vi "Pendel2.vi"() -> ()   [LabVIEW 2014]
uses:
  Reglertyp.ctl
  <vilib>/Platform/TimedLoop/XDataNode/timing_clust.ctl
  <vilib>/Platform/TimedLoop/XDataNode/nitl_modes.ctl
  <vilib>/Platform/TimedLoop/XDataNode/wakeup.ctl
  <vilib>/Analysis/Matrix/Datatypes/RealMatrix.ctl
  <vilib>/Statechart/Common/IntGuid.ctl
  <vilib>/Statechart/Common/DbgID.ctl
  <vilib>/Analysis/baseanly.llb/Real A x B.vi
  Pendel.lvsc/CompanionDiagram.vi
  Pendel.lvsc/CompanionDiagram.vi/21/SC Main.vi
  Pendel.lvsc/Trigger.ctl
  <vilib>/Statechart/Infrastructure/RTStatechart/RunTime SCN.xnode
  Pendel.lvsc/Inputs.ctl
  Pendel.lvsc/Outputs.ctl
  Pendel.lvsc
  <vilib>/Platform/TimedLoop/XDataNode/XDataNode.xnode
  <vilib>/Platform/TimedLoop/XDataNode/XDNodeRunTimeDep.lvlib
  <vilib>/Analysis/NI_AALBase.lvlib
  <vilib>/Analysis/Matrix/NI_Matrix.lvlib
  <vilib>/ptbypt/NI_PtbyPt.lvlib
  <vilib>/Statechart/Common/NI_SC_LVSCCommonFiles.lvlib
panel:
  out "Kraft berechnet 2":cluster{dbl, dbl, dbl, dbl}(graph)
  out "Winkel 1":dbl
  out "Geschwindigkeit":dbl
  out "Position":dbl
  out "Winkel2":dbl
  out "Winkelgeschwindigkeit2":dbl
  out "Winkelgeschwindigkeit1":dbl
  out "Kraft berechnet":cluster{"Kraft (N)":dbl, dbl}(graph)
  out "Schleifendauer":i64(graph)
  in  "Registerkarte":enum32{"Pendel", "S706", "Wegzähler"}(tab)
  in  "Reglertyp":T1
  in  "Positionieren":bool
  out "Kraft (N)":dbl(graph)
  out "Winkel (Grad)":cluster{"Double":dbl, "Double":dbl}(graph)
  in  "Schließen":bool
  in  "Regler anhalten":bool
  in  "Regler starten":bool
  in  "Ruhelage":bool=TRUE
  in  "Pendelaufbau":T2(ring)
  out "Aktueller Zustand":string
  in  "Referenzieren":bool
  in  "Sollposition (mm)":dbl(slide) scale=-500.0..500.0
  out "Position (mm)":T3(graph)
  out "S706 Status (SDO 6041)":T4
  in  "S706 parametrieren":bool
  out "S706":string
  out "Wegzähler (m)":dbl
  out "Wegzähler (m)":dbl(knob)=6.6072914947233965 scale=5000.0..5000000.0
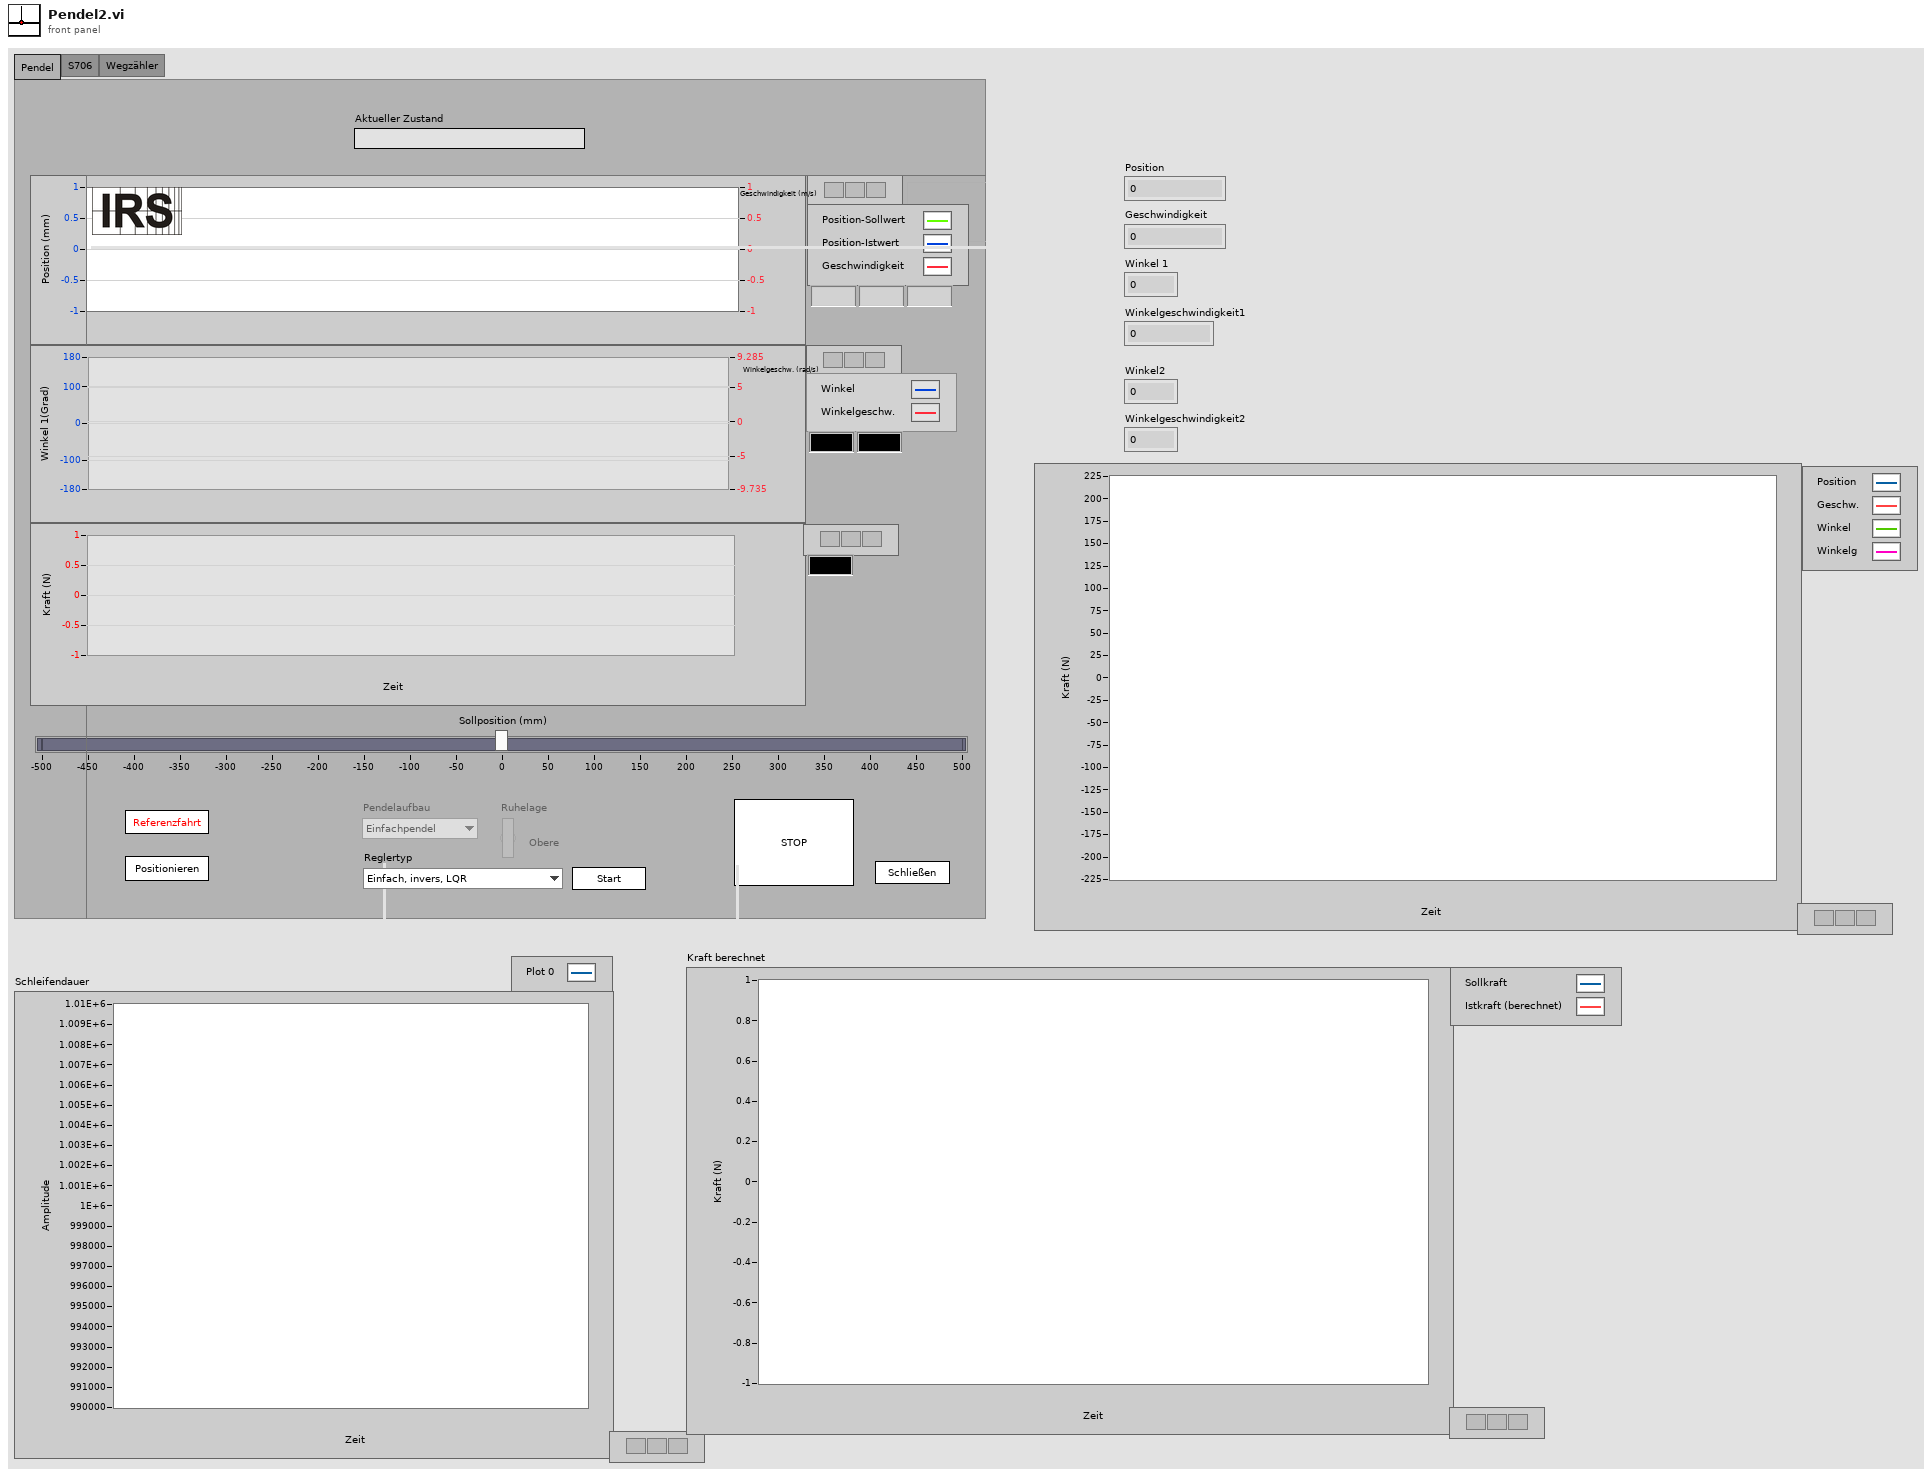
[diagram p1: front panel]
types:
  T1 = typedef "Reglertyp.ctl" = enum16{"Einfach, invers, LQR", "Doppelt, invers, LQR"}
  T2 = enum16{"Einfachpendel", "Doppelpendel", "Dreifachpendel"}
  T3 = cluster{"Sollposition (mm)":dbl, dbl, "Double":dbl}
  T4 = cluster{"0 ready to switch on":bool, "1 switched on":bool, "2 operation enable":bool, "3 fault":bool, "4 voltage enabled":bool, "5 quick stop":bool, "6 switch on disable":bool, "7 warning":bool, "8 ":bool, "9 remote (kann kommunizieren)":bool, "10 target_reached":bool, "11 internal_limit_active":bool, "12 Referenzfahrt durchgeführt":bool, "13 Referenzfahrtfehler":bool}
  T5 = cluster{"Pendelaufbau":enum16{"Einfachpendel", "Doppelpendel", "Dreifachpendel"}, "Winkel1":refnum<k21>, "Winkel2":refnum<k21>, "Winkel3":refnum<k21>}
  T6 = cluster{"node-ID":u8, "RPDO1 controlword":refnum<k20>, "TPDO1 status":refnum<k20>, "RPDO2 I-Sollwert":refnum<k20>, "TPDO2 Ist-Werte":refnum<k20>, "SYNC object":refnum<k20>}
  T7 = typedef "XDNodeRunTimeDep.lvlib/timing_clust.ctl" = cluster{"Expected End [f-1]":u64, "Actual End [f-1]":u64, "Finished Late? [f-1]":bool, "Expected End [i-1]":u64, "Actual End [i-1]":u64, "Finished Late? [i-1]":bool, "Expected Start [i]":u64, "Actual Start [i]":u64, "Expected Start [f]":u64, "Actual Start [f]":u64, "Source Name":string, "Structure Name":string, "Period":i64, "Deadline":i64, "Offset":i64, "Start":i64, "Priority":i32, "Timeout":i32, "Mode":T8, "Wakeup Reason":T9, "Error":errorcluster, "Source Type":string, "Secondary Source Type":string, "Global End Time":u64, "Global Start Time":u64, "Frame Duration":u64, "Iteration Duration":u64, "Assigned CPU":i32, "I/O Scan Engine Mode":u32}
  T8 = typedef "XDNodeRunTimeDep.lvlib/nitl_modes.ctl" = enum32{"No Change", "Process missed periods, maintain original phase", "Discard missed periods, maintain original phase", "Process missed periods, ignore original phase", "Discard missed periods, ignore original phase"}
  T9 = typedef "XDNodeRunTimeDep.lvlib/wakeup.ctl" = enum32{"Normal", "Aborted", "Asynchronous wakeup", "Timing source error", "Timed loop error", "Timeout"}
  T10 = typedef "NI_Matrix.lvlib/RealMatrix.ctl" = dbl[][]
  T11 = cluster{"Winkel1":dbl, "Winkel2":dbl, "Winkel3":dbl}
  T12 = cluster{"Winkelgeschwindigkeit1":dbl, "Winkelgeschwindigkeit2":dbl, "Winkelgeschwindigkeit3":dbl}
  T13 = typedef "NI_SC_LVSCCommonFiles.lvlib/IntGuid.ctl" = cluster{"Data1":u32, "Data2":u16, "Data3":u16, "Data4":u8, "Data5":u8, "Data6":u8, "Data11":u8, "Data9":u8, "Data10":u8, "Data8":u8, "Data7":u8}
  T14 = typedef "NI_SC_LVSCCommonFiles.lvlib/DbgID.ctl" = cluster{"VIRef":u32, "IntGUID":T13}
  T15 = enum16{"unbekannt", "Quick stop active", "Fault reaction active", "Fault", "Operation enabled", "Switched on", "Ready to switch on", "Switch on disabled", "Not Ready to switch on"}
  T16 = cluster{bool, bool, bool, bool, bool, bool, bool, bool, bool, bool, bool, bool, bool, bool}
  T17 = cluster{"Positionieren":bool, "Referenzieren":bool, "Regler darf starten":bool, "Regler anhalten":bool, "Schließen":bool, "S706 parametrieren":bool, "error out":errorcluster}
  T18 = typedef "Pendel.lvsc/Outputs.ctl" = cluster{"Zustand":string, "error out":errorcluster}
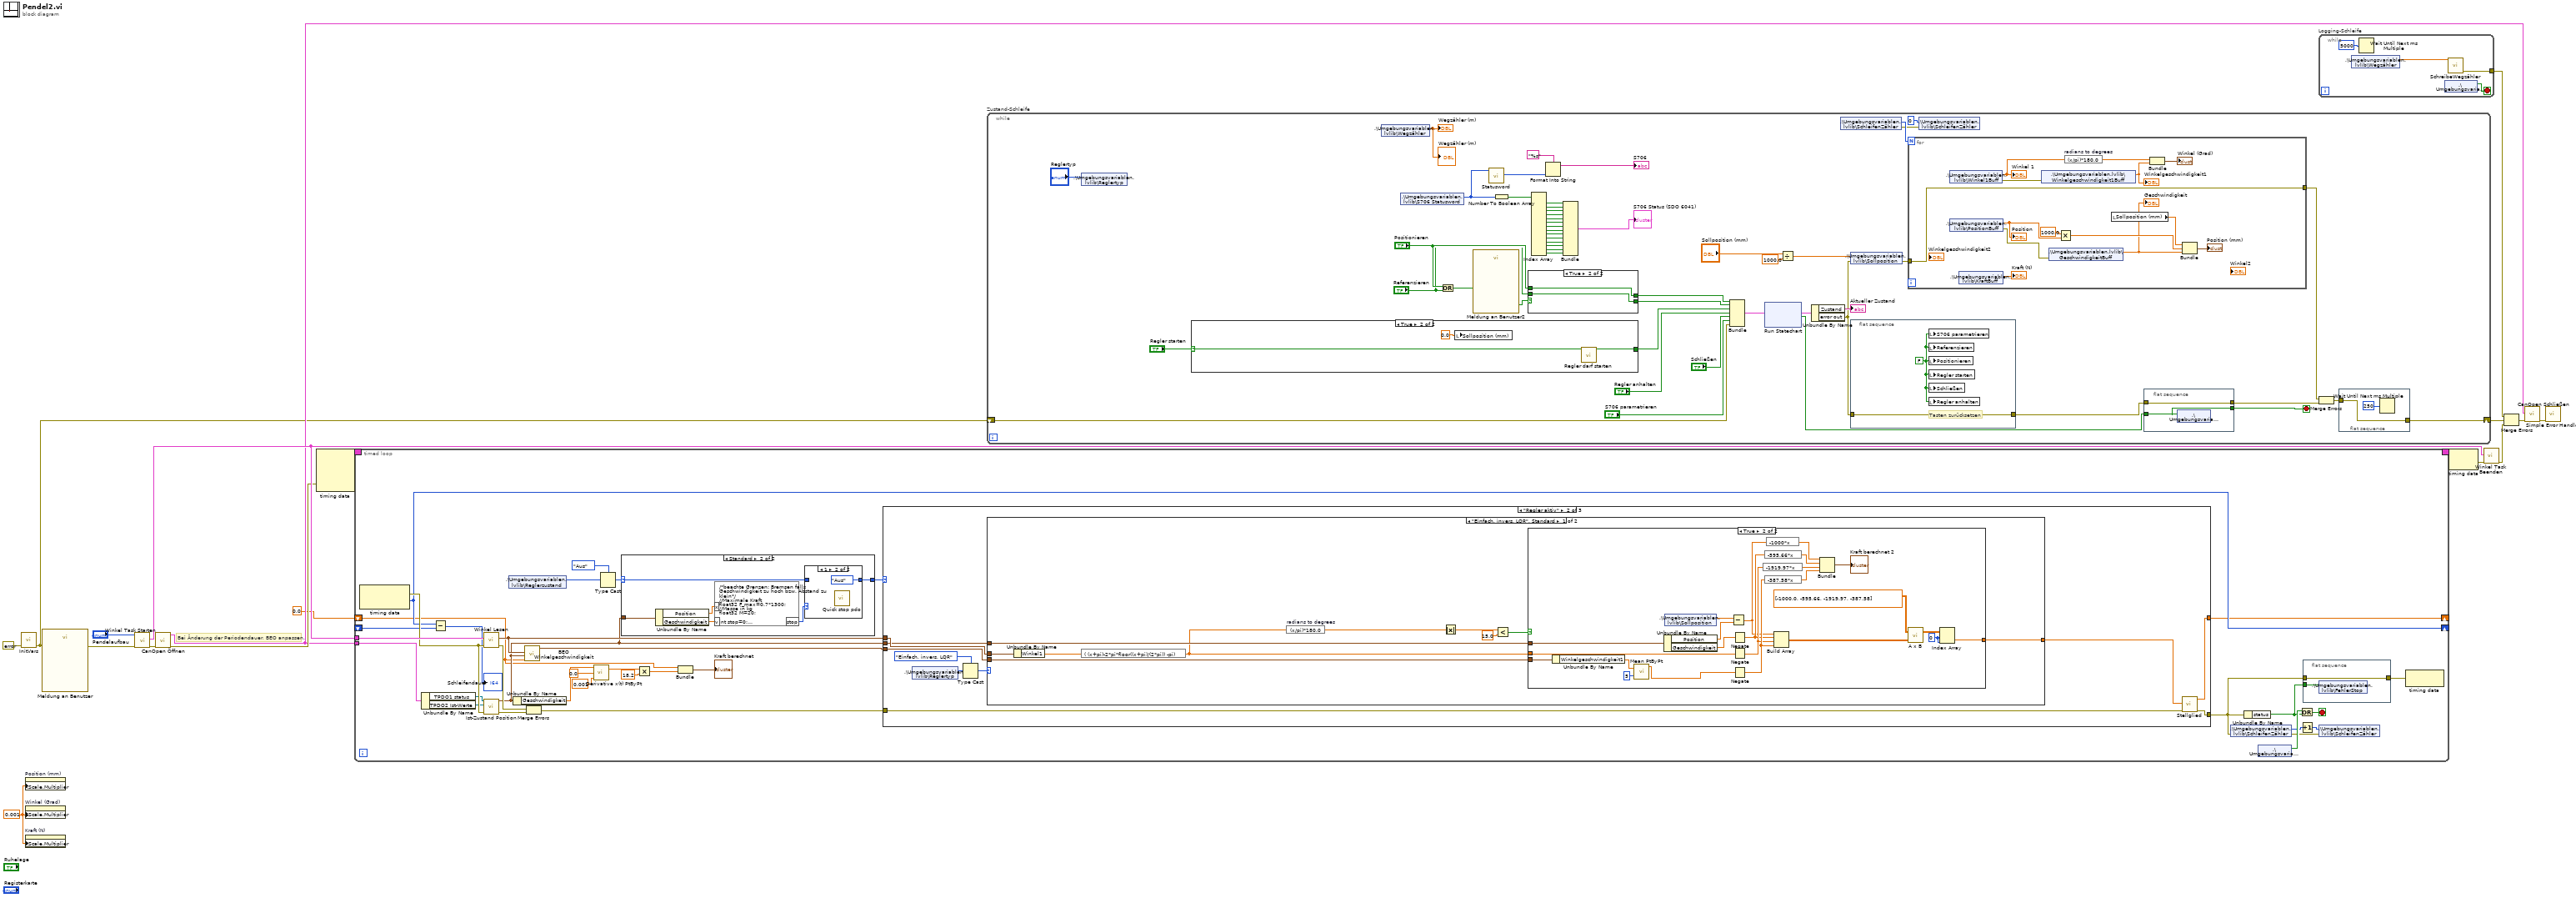
[diagram p0: block diagram]
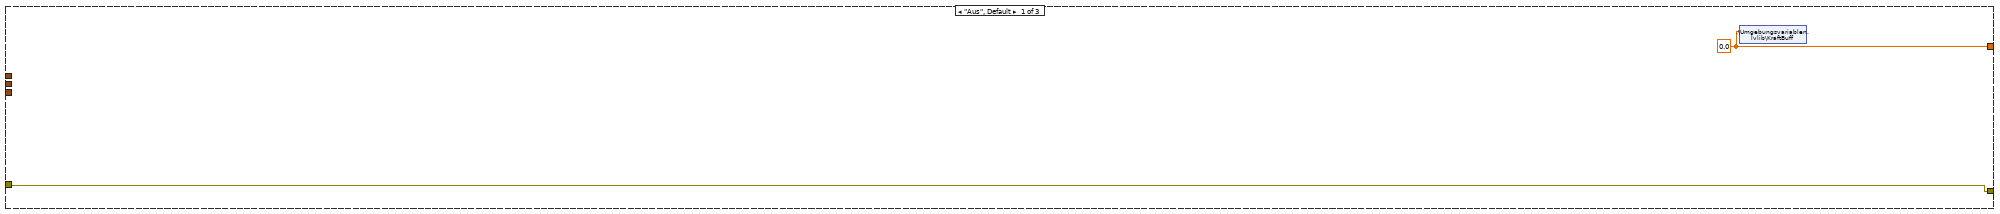
[diagram p4: hidden frame]
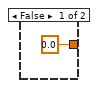
[diagram p5: hidden frame]
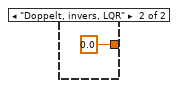
[diagram p6: hidden frame]
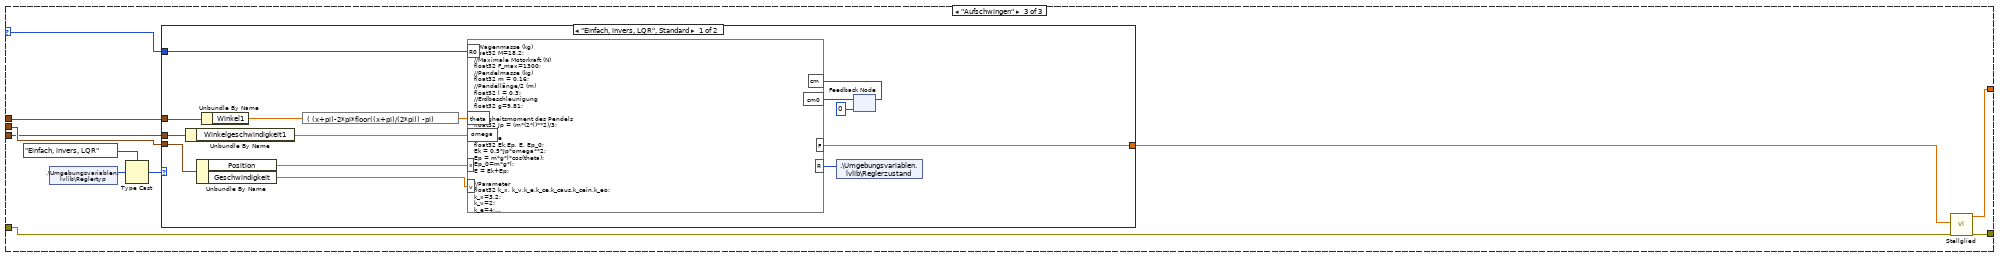
[diagram p7: hidden frame]
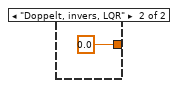
[diagram p8: hidden frame]
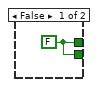
[diagram p9: hidden frame]
diagram:
  w5 = 0.001 ("X-Achse.Offset und Faktor:Faktor")
  # "Bei Änderung der Periodendauer, BEO anpassen."
  n1 = call "InitVars.vi"("error in (no error)"=errorcluster {"status"=FALSE, "code"=0, "source"=""} ("error IO")) -> ("error out"=w4:errorcluster)  [unwired: 10 in]
  n2 = property on="Position (mm)" class="SVDiagr (strikt)"("XScale.Multiplier"=w5) -> ()  [unwired: 2 in, 2 out]
  n3 = property on="Winkel (Grad)" class="SVDiagr (strikt)"("XScale.Multiplier"=w5) -> ()  [unwired: 2 in, 2 out]
  n4 = property on="Kraft (N)" class="SVDiagr (strikt)"("XScale.Multiplier"=w5) -> ()  [unwired: 2 in, 2 out]
  n5 = call "Meldung an Benutzer"("error in (no error)"=w4) -> ("error out"=w10:errorcluster)  [unwired: 9 in, 1 out]
  n6 = call "Winkel Task Starten.vi"("error IO"=w10, "Pendelaufbau in"="Pendelaufbau") -> ("error out"=w2:errorcluster, "Winkel Task"=w13:T5)  [unwired: 8 in]
  n7 = call "CanOpen Öffnen.vi"("error in (no error)"=w2) -> ("Fehler (Ausgang)"=w12:errorcluster, "CanOpen Obj"=w11:T6)  [unwired: 9 in]
  n8 = node-c288(w12) -> (w18:T7)  [unwired: 3 in]
  n9 = timed-loop {
    timing: w18 -> [_]
    timing-out: [_] -> w17
    tunnel: w13 -> [w53]
    tunnel: w11 -> [w48]
    shift-right: [w41] -> _
    shift-left: _ -> [w42]
    shift-right: [w34] -> _
    shift-left: 0.0 ("Kraft (N)") -> [w19]
    stop <- w50 stop-if-true
    n10 = node-c288() -> (w47:errorcluster, w41:i64)  [unwired: 1 in]
    n11 = Unbundle By Name(w48) -> ("TPDO1 status"=w46:refnum<k20>, "TPDO2 Ist-Werte"=w45:refnum<k20>)
    n12 = Subtract(x=w41, y=w42) -> (x-y=→"Schleifendauer":i64)
    n13 = call "Winkel Lesen.vi"("error IO"=w47, "Task In"=w53) -> ("error out"=w43:errorcluster, "Winkel"=w22:T11)  [unwired: 8 in]
    n14 = call "Ist-Zustand Position.vi"("Fehler (Eingang, kein Fehler)"=w47, "TPDO2 object in"=w45, "TPDO1 object in"=w46) -> ("error out"=w44:errorcluster, "Ist-Zustand Position"=w21:cluster{"Position":dbl, "Geschwindigkeit":dbl})  [unwired: 7 in]
    n15 = shared-variable ".\\Umgebungsvariablen.lvlib\\Reglerzustand"() -> (w28:u16)  [unwired: 1 in, 1 out]
    n16 = Unbundle By Name(w21) -> ("Geschwindigkeit"=w30:dbl)
    n17 = call "BEO Winkelgeschwindigkeit.vi"("Kraft (N)"=w19, "Ist-Zustand Position (m, m/s)"=w21, "Winkel (rad)"=w22) -> ("Winkelgeschwindigkeit (1/s)"=w39:T12)  [unwired: 8 in]
    n18 = Merge Errors(w43, w44) -> (w51:errorcluster)
    n19 = call <vilib>:"Derivative x(t) PtByPt.vi"("dt"=0.001, "initial condition"=0.0, "x"=w30) -> ("dx/dt"=w36:dbl)  [unwired: 1 in, 1 out]
    n20 = Type Cast(type=enum16{"Aus", "Aufschwingen", "Regler aktiv"}."Aus", x=w28) -> (*(type *) &x=w24:enum16{"Aus", "Aufschwingen", "Regler aktiv"})
    n21 = case shown="Standard" w24 {
      selector: w24 -> [w54 w56]
      tunnel: [w54 w55] -> w23
      tunnel: w21 -> [_ w60]
      frame "Aus" {
      }
      frame Default {
        n22 = Unbundle By Name(w60) -> ("Position"=w58:dbl, "Geschwindigkeit"=w59:dbl)
        n23 = formula code="/*beachte Grenzen: Bremsen falls Geschwindigkeit zu hoch bzw. Abstand zu klein*/\n//Maximale Kraft\nfloat32 F_max=0.7*1300;\n//Masse in kg\nfloat32 M=20;\n\nint stop=0;\nif((abs(x)+0.5*M/F_max*v**2)>=0.75)\nstop=1;"("x"=w58, "v"=w59) -> ("stop"=w57:i32)
        n24 = case shown="1" w57 {
          tunnel: w56 -> [w61 _]
          tunnel: [w61 enum16{"Aus", "Aufschwingen", "Regler aktiv"}."Aus"] -> w55
          frame 0, Default {
          }
          frame 1 {
            n25 = call "Quick stop pdo.vi"() -> ()  [unwired: 11 in, 1 out]
          }
        }
      }
    }
    n26 = Multiply(x=w36, y=18.2) -> (x*y=w20:dbl)
    n27 = Bundle("Kraft (N)"=w19, w20) -> (→"Kraft berechnet":cluster{"Kraft (N)":dbl, dbl})  [unwired: 1 in]
    n28 = case shown="\"Regler aktiv\"" w23 {
      selector: w23 -> [_ _ w117]
      tunnel: w22 -> [_ w76 w118]
      tunnel: w21 -> [_ w72 w119]
      tunnel: w39 -> [_ w75 w116]
      tunnel: w51 -> [w66 w70 w120]
      tunnel: [w66 w74 w122] -> w26
      tunnel: [w65 w71 w121] -> w34
      frame "Aus", Default {
        w65 = 0.0 ("Kraft (N)")
        n29 = shared-variable ".\\Umgebungsvariablen.lvlib\\KraftBuff"(w65) -> ()  [unwired: 1 in, 1 out]
      }
      frame "Regler aktiv" {
        n30 = shared-variable ".\\Umgebungsvariablen.lvlib\\Reglertyp"() -> (w69:i16)  [unwired: 1 in, 1 out]
        n31 = Type Cast(type=Reglertyp."Einfach, invers, LQR" ("Regler"), x=w69) -> (*(type *) &x=w67:T1)
        n32 = case shown="\"Einfach, invers, LQR\", Standard" w67 {
          tunnel: w76 -> [w86 _]
          tunnel: [w83 0.0 ("Real Matrix Element")] -> w73
          tunnel: w75 -> [w85 _]
          tunnel: w72 -> [w84 _]
          frame "Einfach, invers, LQR", Default {
            n33 = Unbundle By Name(w86) -> ("Winkel1"=w78:dbl)
            n34 = expression code="( (x+pi)-2*pi*floor((x+pi)/(2*pi)) -pi)" ("Ausdrucksknoten")(w78) -> (w77:dbl)
            n35 = expression code="(x/pi)*180.0" "radians to degrees"(w77) -> (w80:dbl)
            n36 = Absolute Value(x=w80) -> (abs(x)=w81:dbl)
            n37 = Less?(x=w81, y=15.0) -> (x < y?=w82:bool)
            n38 = case shown="True" w82 {
              tunnel: w85 -> [_ w110]
              tunnel: w84 -> [_ w109]
              tunnel: w77 -> [_ w108]
              tunnel: [0.0 ("Real Matrix Element") w100] -> w83
              frame False {
              }
              frame True {
                w102 = 0 ("Index (Zeile)")
                n39 = Unbundle By Name(w110) -> ("Winkelgeschwindigkeit1"=w90:dbl)
                n40 = call <vilib>:"Mean PtByPt.vi"("x"=w90, "sample length"=5) -> ("mean"=w89:dbl)  [unwired: 2 in, 1 out]
                n41 = Unbundle By Name(w109) -> ("Position"=w105:dbl, "Geschwindigkeit"=w107:dbl)
                n42 = shared-variable ".\\Umgebungsvariablen.lvlib\\Sollposition"() -> (w106:dbl)  [unwired: 1 in, 1 out]
                n43 = Subtract(x=w106, y=w105) -> (x-y=w91:dbl)
                n44 = Negate(x=w107) -> (-x=w92:dbl)
                n45 = Negate(x=w108) -> (-x=w93:dbl)
                n46 = Negate(x=w89) -> (-x=w97:dbl)
                n47 = expression code="-1919.97*x"(w93) -> (w95:dbl)
                n48 = expression code="-595.66*x"(w92) -> (w94:dbl)
                n49 = expression code="-387.58*x"(w97) -> (w96:dbl)
                n50 = expression code="-1000*x"(w91) -> (w98:dbl)
                n51 = Build Array(w91, w92, w93, w97) -> (w104:T10)
                n52 = Bundle(w98, w94, w95, w96) -> (→"Kraft berechnet 2":cluster{dbl, dbl, dbl, dbl})  [unwired: 1 in]
                n53 = call-poly <vilib>:"A x B.vi"("B"=w104, "A"=T10 [[-1000.0, -595.66, -1919.97, -387.58]]) -> ("A x B"=w101:T10)  [unwired: 1 out]
                n54 = Index Array(array=w101, index (row)=w102, index (col)=w102) -> (element=w100:dbl)
              }
            }
          }
          frame "Doppelt, invers, LQR" {
          }
        }
        n55 = call "Stellglied.vi"("error in (no error)"=w70, "Stellgröße - Kraft (N)"=w73) -> ("error out"=w74:errorcluster, "Kraft (N)"=w71:dbl)  [unwired: 8 in]
      }
      frame "Aufschwingen" {
        n56 = shared-variable ".\\Umgebungsvariablen.lvlib\\Reglertyp"() -> (w114:i16)  [unwired: 1 in, 1 out]
        n57 = Type Cast(type=Reglertyp."Einfach, invers, LQR" ("Regler"), x=w114) -> (*(type *) &x=w112:T1)
        n58 = case shown="\"Einfach, invers, LQR\", Standard" w112 {
          tunnel: w119 -> [w127 _]
          tunnel: w118 -> [w126 _]
          tunnel: w117 -> [w125 _]
          tunnel: w116 -> [w124 _]
          tunnel: [w123 sgl 0.0] -> w115
          frame "Einfach, invers, LQR", Default {
            n59 = Unbundle By Name(w124) -> ("Winkelgeschwindigkeit1"=w135:dbl)
            n60 = Unbundle By Name(w127) -> ("Position"=w134:dbl, "Geschwindigkeit"=w136:dbl)
            n61 = Unbundle By Name(w126) -> ("Winkel1"=w132:dbl)
            n62 = expression code="( (x+pi)-2*pi*floor((x+pi)/(2*pi)) -pi)" ("Ausdrucksknoten")(w132) -> (w133:dbl)
            n63 = feedback #1 ("Rückkopplungsknoten")(0) -> (w129:i32)
            n64 = formula code="//Wagenmasse (kg)\nfloat32 M=18.2;\n//Maximale Motorkraft (N)\nfloat32 F_max=1300;\n//Pendelmasse (kg)\nfloat32 m = 0.16; \n//Pendellänge/2 (m)\nfloat32 l = 0.3; \n//Erdbeschleunigung\nfloat32 g=9.81;\n\n//Trägheitsmoment des Pendels\nfloat32 Jp = (m*(2*l)**2)/3;\n\n//Energie\nfloat32 Ek,Ep, E, Ep_0;\nEk = 0.5*Jp*omega**2;\nEp = m*g*l*cos(theta);\nEp_0=m*g*l;\nE = Ek+Ep;\n\n//Parameter\nfloat32 k_x, k_v,k_e,k_ce,k_caus,k_cein,k_eo;\nk_x=3.2;\nk_v=2;\nk_e=4;\nk_ce=4;\nk_caus=0.75;\nk_cein=1;\nk_eo=1;\n//k_eo=1.05;\n\n//Potentialtopf - Position\nfloat32 u_x;\nif(abs(x)<0.6)\nu_x=k_x*sign(x)*ln(1-abs(x)/0.6);\nelse\nu_x=-F_max/M*sign(x);\n\n//Potentialtopf - Geschwindigkeit\nfloat32 u_v;\nif(abs(v)<6)\nu_v=k_v*sign(v)*ln(1-abs(v)/6);\nelse\nu_v=-F_max/M*sign(v);\n\nint cm;\nif(E>k_cein*Ep_0) \ncm=1;\nelse if (E<k_caus*Ep_0) \ncm=0;\nelse\ncm=cm0;\n\nfloat32 u, F;\nif(cm)\nu=u_x + u_v+k_ce*(E-k_eo*Ep_0)*sign(omega*cos(theta));\n//u=u_x + u_v+k_ce*(exp(abs(E-k_eo*Ep_0))-1)*sign(E-Ep_0)*sign(omega*cos(theta));\nelse\nu=-k_e*sign(omega*cos(theta))+u_x;\nu=2*u;\nF=(Jp*(M+m)-(m*l)**2*cos(theta)**2)/Jp*u-m*l*sin(theta)*omega**2+(m*l)**2*g*sin(theta)*cos(theta)/Jp;\n\n/*Regler aktivieren?*/\nint R=1; //Regelzustand: Aufschwingen\nif( abs(theta)/pi*180<10 && abs(x)<0.4 && abs(omega)<1 || (R0==1 &&abs(theta)/pi*180<15))\nR=2; //Reglerzustand: Regler aktiviert"("x"=w134, "v"=w136, "theta"=w133, "omega"=w135, "cm0"=w129, "R0"=w125) -> ("F"=w123:sgl, "cm"=w128:i32, "R"=w131:i32)
            n65 = shared-variable ".\\Umgebungsvariablen.lvlib\\Reglerzustand"(w131) -> ()  [unwired: 1 in, 1 out]
            n66 = feedback-in #1 ("2")(w128) -> ()
          }
          frame "Doppelt, invers, LQR" {
          }
        }
        n67 = call "Stellglied.vi"("error in (no error)"=w120, "Stellgröße - Kraft (N)"=w115) -> ("error out"=w122:errorcluster, "Kraft (N)"=w121:dbl)  [unwired: 8 in]
      }
    }
    n68 = shared-variable ".\\Umgebungsvariablen.lvlib\\SchleifenZähler"(error in=w26) -> (w32:u16, error out=w31:errorcluster)
    n69 = Unbundle By Name(w26) -> ("status"=w27:bool)
    n70 = shared-variable ".\\Umgebungsvariablen.lvlib\\stop"() -> (w49:bool)  [unwired: 1 in, 1 out]
    n71 = Or(x=w49, y=w27) -> (x .or. y?=w50:bool)
    n72 = Increment(x=w32) -> (x+1=w33:u16)
    n73 = flat-sequence {
      tunnel: w27 -> [w64]
      tunnel: w26 -> [w63]
      tunnel: [w63] -> w25
      frame #0 {
        n74 = shared-variable ".\\Umgebungsvariablen.lvlib\\FehlerStop"(w64) -> ()  [unwired: 1 in, 1 out]
      }
    }
    n75 = shared-variable ".\\Umgebungsvariablen.lvlib\\SchleifenZähler"(w33, error in=w31) -> ()  [unwired: 1 out]
    n76 = node-c288(w25) -> ()  [unwired: 1 out]
  }
  n77 = while "Zustand-Schleife" {
    shift-right: [w187] -> w16
    shift-left: w4 -> [w168]
    stop <- w189 stop-if-true
    n78 = shared-variable ".\\Umgebungsvariablen.lvlib\\Reglertyp"("Reglertyp") -> ()  [unwired: 1 in, 1 out]
    n79 = case shown="True" "Regler starten" {
      selector: "Regler starten" -> [w199 w201]
      tunnel: [w199 w200] -> w152
      frame False {
      }
      frame True {
        n80 = local write "Sollposition (mm)"(0.0 ("Sollposition (mm)")) -> ()
        n81 = call "Regler darf starten.vi"("Regler start"=w201) -> ("Regler darf starten"=w200:bool)  [unwired: 10 in]
      }
    }
    n82 = shared-variable ".\\Umgebungsvariablen.lvlib\\Wegzähler"() -> (→"Wegzähler (m)" →"Wegzähler (m)":dbl)  [unwired: 1 in, 1 out]
    n83 = shared-variable ".\\Umgebungsvariablen.lvlib\\S706 Statusword"() -> (w184:u16)  [unwired: 1 in, 1 out]
    n84 = Or(x="Positionieren", y="Referenzieren") -> (x .or. y?=w151:bool)
    n85 = call "Meldung an Benutzer2"("Enable"=w151) -> ("OK"=w150:bool)  [unwired: 9 in, 1 out]
    n86 = call "Statusword.vi"("Wert"=w184) -> ("Status"=w159:T15)  [unwired: 10 in]
    n87 = Number To Boolean Array(number=w184) -> (Boolean array=w185:bool[])
    n88 = case shown="True" w150 {
      tunnel: "Referenzieren" -> [_ w197]
      tunnel: "Positionieren" -> [_ w198]
      tunnel: [w196 w198] -> w148
      tunnel: [w196 w197] -> w146
      frame False {
        w196 = FALSE ("Positionieren")
      }
      frame True {
      }
    }
    n89 = Index Array(array=w185) -> (element #1=w183:bool, element #2=w182:bool, element #3=w181:bool, element #4=w180:bool, element #5=w179:bool, element #6=w178:bool, element #7=w177:bool, element #8=w176:bool, element #9=w175:bool, element #10=w174:bool, element #11=w173:bool, element #12=w172:bool, element #13=w171:bool, element #14=w170:bool)  [unwired: 14 in]
    n90 = Format Into String(format string="%s" ("Format-String"), w159) -> (resulting string=→"S706":string)  [unwired: 2 in, 1 out]
    n91 = Bundle(w183, w182, w181, w180, w179, w178, w177, w176, w175, w174, w173, w172, w171, w170) -> (→"S706 Status (SDO 6041)":T16)  [unwired: 1 in]
    n92 = Bundle("Positionieren"=w148, "Referenzieren"=w146, "Regler darf starten"=w152, "Regler anhalten"="Regler anhalten", "Schließen"="Schließen", "S706 parametrieren"="S706 parametrieren", "error out"=w168) -> (w190:T17)  [unwired: 1 in]
    n93 = xnode "Run Statechart"("Inputs"=w190) -> ("Terminated?"=w191:bool, "Outputs"=w193:T18)  [unwired: 2 in]
    n94 = Divide(x="Sollposition (mm)", y=1000.0) -> (x/y=w162:dbl)
    n95 = Unbundle By Name(w193) -> ("Zustand"=→"Aktueller Zustand":string, "error out"=w153:errorcluster)
    n96 = shared-variable ".\\Umgebungsvariablen.lvlib\\SchleifenZähler"() -> (w165:u16, error out=w163:errorcluster)  [unwired: 1 in]
    n97 = shared-variable ".\\Umgebungsvariablen.lvlib\\Sollposition"(w162, error in=w153) -> (error out=w154:errorcluster)
    n98 = flat-sequence {
      tunnel: [w222] -> w166
      tunnel: w153 -> [w222]
      frame #0 {
        w221 = FALSE
        # "Tasten zurücksetzen"
        n99 = local write "S706 parametrieren"(w221) -> ()
        n100 = local write "Referenzieren"(w221) -> ()
        n101 = local write "Positionieren"(w221) -> ()
        n102 = local write "Regler starten"(w221) -> ()
        n103 = local write "Schließen"(w221) -> ()
        n104 = local write "Regler anhalten"(w221) -> ()
      }
    }
    n105 = for {
      N: w165 -> [_]
      tunnel: w154 -> [w208]
      tunnel: [w208] -> w167
      n106 = shared-variable ".\\Umgebungsvariablen.lvlib\\Winkel1Buff"() -> (w210:dbl, error out=w211:errorcluster)  [unwired: 1 in]
      "Winkel 1" <- w210
      n107 = shared-variable ".\\Umgebungsvariablen.lvlib\\PositionBuff"() -> (w213:dbl, error out=w207:errorcluster)  [unwired: 1 in]
      "Position" <- w213
      n108 = shared-variable ".\\Umgebungsvariablen.lvlib\\KraftBuff"() -> (→"Kraft (N)":dbl)  [unwired: 1 in, 1 out]
      n109 = shared-variable ".\\Umgebungsvariablen.lvlib\\Winkelgeschwindigkeit1Buff"(error in=w211) -> (w203:dbl)  [unwired: 1 out]
      "Winkelgeschwindigkeit1" <- w203
      n110 = shared-variable ".\\Umgebungsvariablen.lvlib\\GeschwindigkeitBuff"(error in=w207) -> (w205:dbl)  [unwired: 1 out]
      "Geschwindigkeit" <- w205
      n111 = Multiply(x=1000.0, y=w213) -> (x*y=w215:dbl)
      n112 = expression code="(x/pi)*180.0" "radians to degrees"(w210) -> (w206:dbl)
      n113 = local read "Sollposition (mm)"() -> (w204:dbl)
      n114 = Bundle("Double"=w206, "Double"=w203) -> (→"Winkel (Grad)":cluster{"Double":dbl, "Double":dbl})  [unwired: 1 in]
      n115 = Bundle("Sollposition (mm)"=w204, w215, "Double"=w205) -> (→"Position (mm)":T3)  [unwired: 1 in]
    }
    n116 = shared-variable ".\\Umgebungsvariablen.lvlib\\SchleifenZähler"(u16 0 ("SchleifenZähler"), error in=w163) -> ()  [unwired: 1 out]
    n117 = flat-sequence {
      tunnel: w166 -> [w219]
      tunnel: [w219] -> w156
      tunnel: w191 -> [w220]
      tunnel: [w220] -> w189
      frame #0 {
        n118 = shared-variable ".\\Umgebungsvariablen.lvlib\\stop"(w220) -> ()  [unwired: 1 in, 1 out]
      }
    }
    n119 = Merge Errors(w167, w156) -> (w188:errorcluster)
    n120 = flat-sequence {
      tunnel: [w218] -> w187
      tunnel: w188 -> [w218]
      frame #0 {
        n121 = Wait Until Next ms Multiple(millisecond multiple=u32 250 ("ms")) -> ()  [unwired: 1 out]
      }
    }
  }
  n122 = while "Logging-Schleife" {
    tunnel: [w242] -> w1
    stop <- w240 stop-if-true
    n123 = shared-variable ".\\Umgebungsvariablen.lvlib\\Wegzähler"() -> (w243:dbl)  [unwired: 1 in, 1 out]
    n124 = Wait Until Next ms Multiple(millisecond multiple=u32 5000 ("ms")) -> ()  [unwired: 1 out]
    n125 = shared-variable ".\\Umgebungsvariablen.lvlib\\stop"() -> (w240:bool)  [unwired: 1 in, 1 out]
    n126 = call "SchreibeWegzähler.vi"("Aktuell"=w243) -> ("error out"=w242:errorcluster)  [unwired: 10 in]
  }
  n127 = node-c288(w17) -> (w15:errorcluster)
  n128 = call "Winkel Task Beenden.vi"("error IO"=w15, "Task In"=w13) -> ("error out"=w8:errorcluster)  [unwired: 9 in]
  n129 = Merge Errors(w1, w16, w8) -> (w7:errorcluster)
  n130 = call "CanOpen Schließen.vi"("error in (no error)"=w7, "CanOpen Obj"=w11) -> ("Fehler (Ausgang)"=w6:errorcluster)  [unwired: 9 in]
  n131 = call <vilib>:"Simple Error Handler.vi"("error in (no error)"=w6) -> ()  [unwired: 4 in, 5 out]
